vi "Unpack Winbounds.vi"(3 "value":string) -> (1 "Front Panel.WinBounds":T1)   [LabVIEW 2015, in "User Interface.lvlib"]
uses:
  User Interface.lvlib
  <vilib>/Utility/miscctls.llb/LVRectTypeDef.ctl
  Error Correction/Error Correction.lvlib
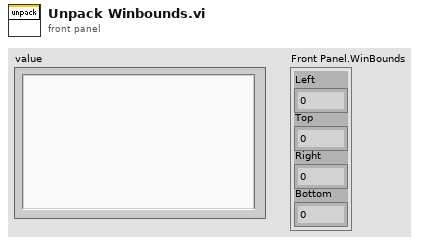
[diagram p1: front panel]
types:
  T1 = typedef "LVRectTypeDef.ctl" = cluster{"Left":i16, "Top":i16, "Right":i16, "Bottom":i16}
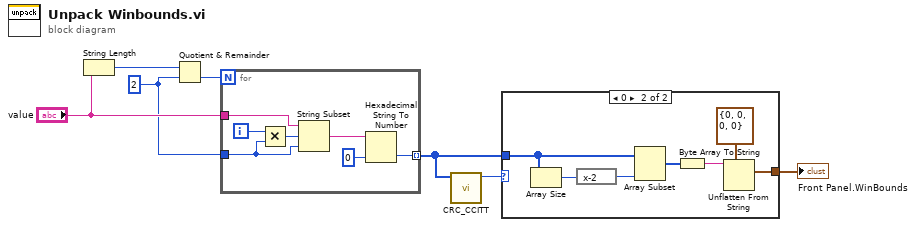
[diagram p0: block diagram]
diagram:
  w2 = 2 ("length (rest)")
  n1 = String Length(string="value") -> (length=w3:i32)
  n2 = Quotient & Remainder(x=w3, y=w2) -> (floor(x/y)=w4:i32)  [unwired: 1 out]
  n3 = for {
    N: w4 -> [_]
    tunnel: "value" -> [w14]
    tunnel: [w10] -> w6 mode=indexing
    tunnel: w2 -> [w9]
    i -> [w13]
    n4 = Multiply(x=w13, y=w9) -> (x*y=w12:i32)
    n5 = String Subset(string=w14, offset (0)=w12, length (rest)=w9) -> (substring=w11:string)
    n6 = Hexadecimal String To Number(string=w11, default (0uL)=u8 0 ("default (0 U32)")) -> (number=w10:u8)  [unwired: 1 in, 1 out]
  }
  n7 = call "CRC_CCITT.vi"("unsigned byte array"=w6) -> ("CRC-CCITT"=w1:u16)  [unwired: 5 in, 1 out]
  n8 = case shown="0" w1 {
    tunnel: w6 -> [_ w21]
    tunnel: [_ w15] -> w7
    frame Default {
    }
    frame 0 {
      n9 = Array Size(array=w21) -> (size(s)=w20:i32)
      n10 = expression code="x-2"(w20) -> (w19:i32)
      n11 = Array Subset(array=w21, length=w19) -> (w18:u8[])  [unwired: 1 in]
      n12 = Byte Array To String(unsigned byte array=w18) -> (string=w17:string)
      n13 = Unflatten From String(type=T1 {"Left"=0, "Top"=0, "Right"=0, "Bottom"=0} ("Front Panel.WinBounds"), binary string=w17) -> (value=w15:T1)  [unwired: 3 in, 2 out]
    }
  }
  "Front Panel.WinBounds" <- w7
